vi "resonant.scan.engine.8or12kHz5ch_MD.vi"() -> ()   [LabVIEW 2012]
uses:
  <vilib>/Utility/VariantDataType/Type.ctl
  GFG/GFGbooleanGet.vi
  GFG/GFGnumericGet.vi
  GFG/GFGfpRefGet.vi
  <vilib>/Utility/error.llb/Error Cluster From Error Code.vi
  <vilib>/RVI Host/nirviSupport.llb/nirviErrorClusterFromErrorCode.vi
  <vilib>/rvi/errors/niLvFpgaAdjustHostInterfaceError.vi
  <vilib>/FPGAPlugInAG/PXIe-7962R/niLvFpga_Abort_PXIe-7962R.vi
  <vilib>/FPGAPlugInAG/PXIe-7962R/niLvFpga_Close_PXIe-7962R.vi
  <vilib>/rvi/interface/nirviMethod/nirviMethod.xnode
  FPGA/current bitfiles/4chresonancescan_PXIe-7962R_5ch8or12kHzreson_gAN2W9JJOBI.lvbitx
  <vilib>/rvi/interface/nirviCloseFPGA/nirviCloseFPGA.xnode
  GFG/GFG library.lvlib
  <vilib>/Utility/VariantDataType/VariantType.lvlib
  <vilib>/rvi/errors/niLvFpgaMergeErrorWithErrorCode.vi
  <vilib>/FPGAPlugInAG/PXIe-7962R/niLvFpga_AcknowledgeIrq_PXIe-7962R.vi
  <vilib>/rvi/interface/nirviMethod/StockFPGA_InlinedMethodWaitForSingleIRQ.vi
  <vilib>/FPGAPlugInAG/PXIe-7962R/niLvFpga_WaitOnIrq_PXIe-7962R.vi
  <vilib>/FPGAPlugInAG/PXIe-7962R/niLvFpga_ReadFifo_PXIe-7962R.vi
panel:
  out "x/y":dbl format="%#_6f"
  out "max Elements Remaining 2":u32
  out "Array":i16[][][](array[numeric])
  out "size(s)":i32[](array[numeric])
  out "Elements Remaining":u32
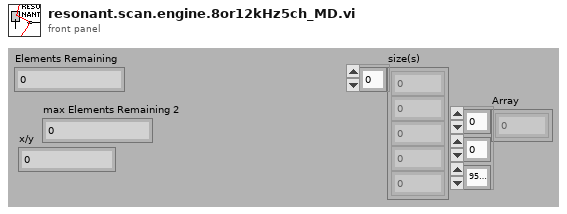
[diagram p1: front panel]
types:
  T1 = enum8{"Enabled", "Disabled", "Disabled and Grayed Out"}
  T2 = cluster{"WaveformChartRef":refnum<vi>, "DigitalRef":refnum<vi>, "ArrayRef":refnum<vi>, "TabControlRef":refnum<vi>, "EnumRef":refnum<vi>, "RingRef":refnum<vi>, "BooleanRef":refnum<vi>, "KnobRef":refnum<vi>, "SlideRef":refnum<vi>, "PathRef":refnum<vi>, "StringRef":refnum<vi>, "ComboBox":refnum<vi>, "WaveformGraphRef":refnum<vi>}
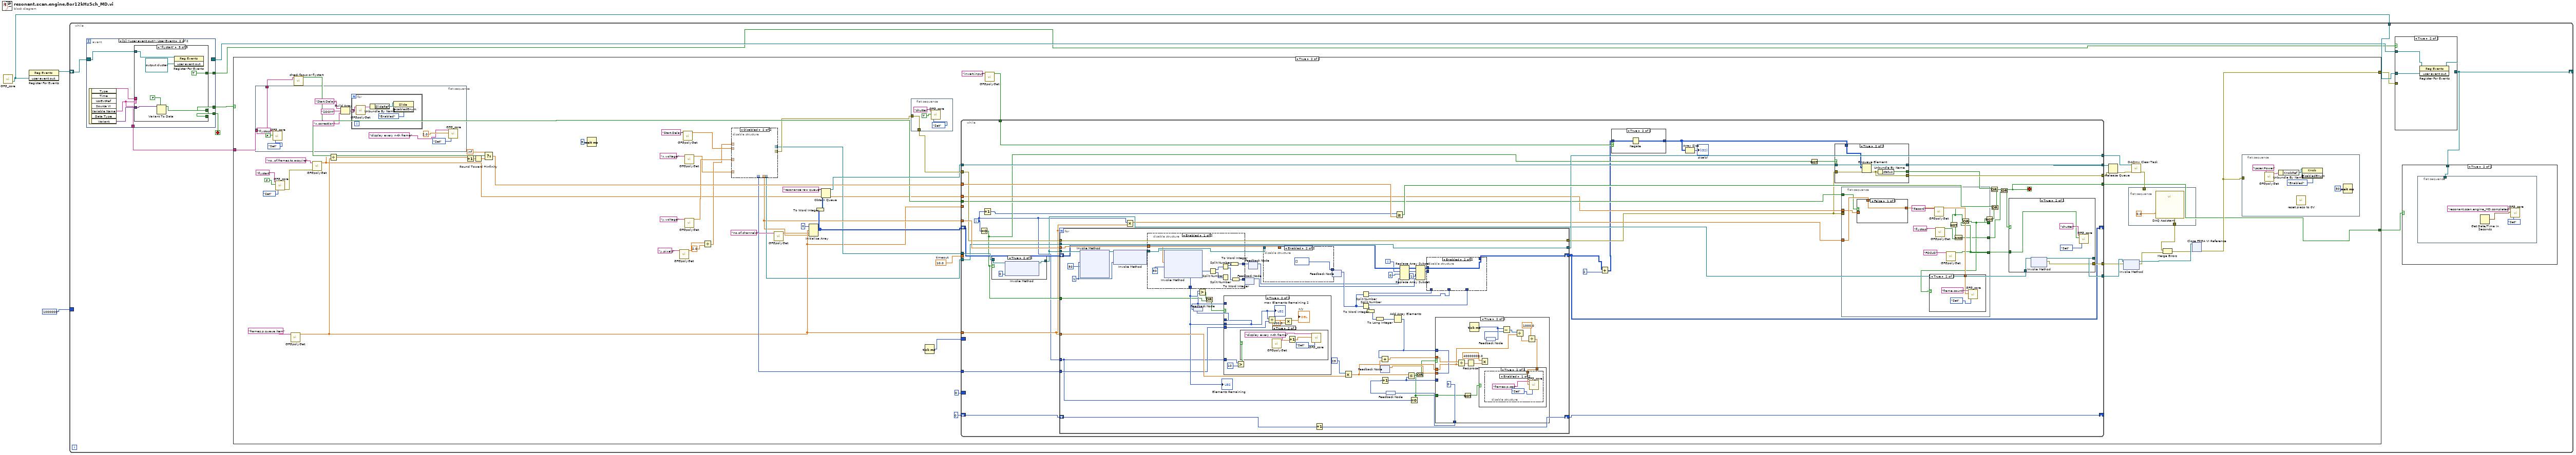
[diagram p0: block diagram]
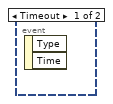
[diagram p4: hidden frame]
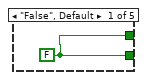
[diagram p5: hidden frame]
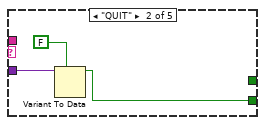
[diagram p6: hidden frame]
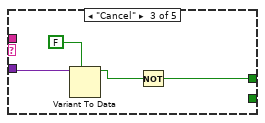
[diagram p7: hidden frame]
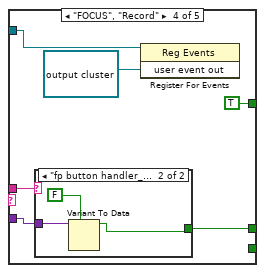
[diagram p8: hidden frame]
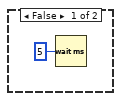
[diagram p10: hidden frame]
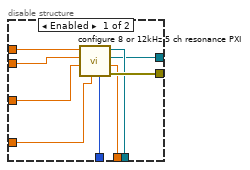
[diagram p11: hidden frame]
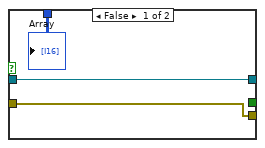
[diagram p12: hidden frame]
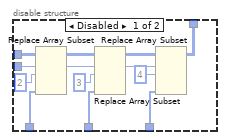
[diagram p13: hidden frame]
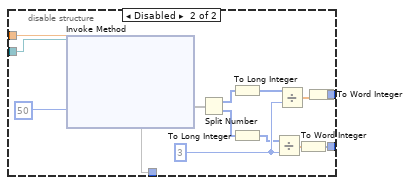
[diagram p14: hidden frame]
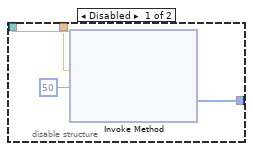
[diagram p15: hidden frame]
diagram:
  n1 = call "GFG_core.vi"() -> ("user event out"=w2:refnum<user-event>)  [unwired: 13 in, 6 out]
  n2 = register-events(w2) -> (reference out=w3:refnum<event-registration>)  [unwired: 2 in, 1 out]
  n3 = while {
    shift-right: [w4] -> _
    shift-left: w3 -> [w11]
    tunnel: w2 -> [w10]
    border: u32 1000000 ("Elements Remaining") -> [_]
    stop <- w12 stop-if-true
    n4 = event shown="[1] <user event out>: User Event" {
      selector: w11 -> [_ w24]
      dyn-events: [_ _] -> w8
      timeout: _ -> [_ _]
      tunnel: [_ w28] -> w13
      tunnel: [_ w27] -> w12
      tunnel: [_ w23] -> w7
      tunnel: [_ w22] -> w6
      event Timeout {
        n5 = event-data() -> ()  [unwired: 1 in, 2 out]
      }
      event User Event {
        n6 = event-data() -> ("Source VI"=w25:string, "Variable Name"=w22:string, "Variant"=w26:variant)  [unwired: 1 in, 4 out]
        n7 = case shown="\"flystart\"" w22 {
          tunnel: [w29 _ w33 w41 w46] -> w28
          tunnel: [w29 w30 _ _ _] -> w27
          tunnel: w26 -> [_ w32 w35 w42 w50]
          tunnel: w25 -> [_ _ _ w40 _]
          tunnel: w24 -> [_ _ _ w38 w47]
          tunnel: [_ _ _ TRUE TRUE] -> w23
          frame "False", Default {
            w29 = FALSE ("NewVal")
          }
          frame "QUIT" {
            n8 = Variant To Data(type=FALSE ("NewVal"), Variant=w32) -> (data=w30:bool)  [unwired: 1 in, 1 out]
          }
          frame "Cancel" {
            n9 = Variant To Data(type=FALSE ("NewVal"), Variant=w35) -> (data=w34:bool)  [unwired: 1 in, 1 out]
            n10 = Not(x=w34) -> (.not. x?=w33:bool)
          }
          frame "FOCUS", "Record" {
            n11 = case shown="\"fp button handler_MD.vi\"" w40 {
              tunnel: w42 -> [_ w44]
              tunnel: [_ w43] -> w41
              frame "False", Default {
              }
              frame "fp button handler_MD.vi" {
                n12 = Variant To Data(type=FALSE ("NewVal"), Variant=w44) -> (data=w43:bool)  [unwired: 1 in, 1 out]
              }
            }
            n13 = register-events(reference=w38, refnum<user-event> refnum ("user event out")) -> ()  [unwired: 1 in, 2 out]
          }
          frame "flystart" {
            n14 = Variant To Data(type=FALSE ("NewVal"), Variant=w50) -> (data=w46:bool)  [unwired: 1 in, 1 out]
            n15 = register-events(reference=w47, refnum<user-event> refnum ("user event out")) -> ()  [unwired: 1 in, 2 out]
          }
        }
      }
    }
    n16 = case shown="True" w13 {
      tunnel: [_ w88] -> w9
      tunnel: w6 -> [_ w56]
      tunnel: [_ w78] -> w5
      frame False {
        n17 = Wait (ms)(milliseconds to wait=u32 5) -> ()  [unwired: 1 out]
      }
      frame True {
        w109 = 10.0  # timeout
        n18 = flat-sequence {
          tunnel: w56 -> [w129]
          tunnel: [w129] -> w55
          frame #0 {
            n19 = call "GFG_core.vi"("Variable Name in"="flystop", "Variant in"=FALSE ("Boolean"), "Action"=enum16{"Init", "Set", "Get"}."Set") -> ()  [unwired: 10 in, 7 out]
            n20 = Build Array("Start.Delay" ("Variable Name in"), "ZOOM" ("Variable Name in"), "x.correction" ("Variable Name in")) -> (w124:string[])
            n21 = for {
              tunnel: w124 -> [w132] mode=indexing
              n22 = call-poly "GFGpolyGet.vi"("Variable Name in"=w132) -> ("output cluster"=w135:T2)  [unwired: 9 in, 1 out]
              n23 = Unbundle By Name(w135) -> ("SlideRef"=w133:refnum<vi>)
              n24 = property class="Slide"(reference=w133, "DisabledEnum"=T1."Enabled" ("Disabled")) -> ()  [unwired: 1 in, 2 out]
            }
            n25 = call "GFG_core.vi"("Variable Name in"="display every n-th frame" ("Tag in"), "Variant in"=2.0 ("Numeric"), "Action"=enum16{"Init", "Set", "Get"}."Set") -> ()  [unwired: 10 in, 7 out]
          }
        }
        n26 = call "GFG_core.vi"("Variable Name in"="flystart" ("Tag in"), "Variant in"=FALSE, "Action"=enum16{"Init", "Set", "Get"}."Set") -> ("error out"=w79:errorcluster)  [unwired: 10 in, 6 out]
        n27 = call-poly "GFGpolyGet.vi"("Variable Name in"="frames.p.queue.item" ("Tag in")) -> ("Numeric"=w61:dbl)  [unwired: 9 in, 1 out]
        n28 = call "check focus or flystart.vi"("x"=w55) -> ("x .or. y?"=w84:bool)  [unwired: 10 in]
        n29 = call-poly "GFGpolyGet.vi"("error in (no error)"=w79, "Variable Name in"="no..of.frames.to.acquire" ("Tag in")) -> ("Numeric"=w60:dbl)  [unwired: 8 in, 1 out]
        n30 = Divide(x=w60, y=w61) -> (x/y=w62:dbl)
        n31 = Increment(x=w62) -> (x+1=w57:dbl)
        n32 = Round Toward +Infinity(x=w57) -> (ceil(x): smallest int >= x=w59:dbl)
        n33 = Select(t=inf, s=w84, f=w59) -> (s? t:f=w85:dbl)
        n34 = Wait (ms)(milliseconds to wait=u32 5) -> ()  [unwired: 1 out]
        n35 = call-poly "GFGpolyGet.vi"("Variable Name in"="y.pixels" ("Tag in")) -> ("Numeric"=w103:dbl)  [unwired: 9 in, 1 out]
        n36 = call-poly "GFGpolyGet.vi"("Variable Name in"="Start.Delay" ("Tag in")) -> ("Numeric"=w75:dbl)  [unwired: 9 in, 1 out]
        n37 = call-poly "GFGpolyGet.vi"("Variable Name in"="x.voltage" ("Tag in")) -> ("Numeric"=w72:dbl)  [unwired: 9 in, 1 out]
        n38 = call-poly "GFGpolyGet.vi"("Variable Name in"="y.voltage" ("Tag in")) -> ("Numeric"=w74:dbl)  [unwired: 9 in, 1 out]
        n39 = Divide(x=w103, y=2.0 ("x")) -> (x/y=w73:dbl)
        n40 = disable-structure shown="Disabled" {
          disable-tunnel: w75 -> [w120 _]
          disable-tunnel: w74 -> [w119 _]
          disable-tunnel: w73 -> [w118 _]
          disable-tunnel: w72 -> [w117 _]
          disable-tunnel: [w116 _] -> w71
          disable-tunnel: [w115 _] -> w70
          disable-tunnel: [w114 _] -> w66
          disable-tunnel: [w112 _] -> w65
          disable-tunnel: [w113 _] -> w63
          frame Enabled {
            n41 = call "configure 8 or 12kHz 5 ch resonance PXI.vi"("x resonant zoom voltage"=w117, "y-voltage"=w119, "Start Delay (Ticks)"=w120, "lines (2pi) per frame"=w118) -> ("error out"=w116:errorcluster, "pixels per frame"=w114:dbl, "FPGA VI Reference Out"=w112:refnum<k20>, "AO task out"=w115:refnum<k21>, "Actual Depth 3"=w113:u32)  [unwired: 3 in]
          }
          frame Disabled {
          }
        }
        n42 = call-poly "GFGpolyGet.vi"("Variable Name in"="no.of.channels" ("Tag in")) -> ("Numeric"=w69:dbl)  [unwired: 9 in, 1 out]
        n43 = Initialize Array(i16 0, w61, w69, w66) -> (w95:i16[][][])
        n44 = To Word Integer(number=w95) -> (16bit integer=w53:i16[][][])
        n45 = Obtain Queue(name (unnamed)="resonance raw queue", element data type=w53) -> (queue out=w96:refnum<queue>)  [unwired: 3 in, 2 out]
        n46 = flat-sequence {
          tunnel: [w143] -> w105
          tunnel: w71 -> [w143]
          frame #0 {
            n47 = call "GFG_core.vi"("Variable Name in"="shutter" ("Tag in"), "Variant in"=TRUE, "Action"=enum16{"Init", "Set", "Get"}."Set") -> ()  [unwired: 10 in, 7 out]
          }
        }
        n48 = Tick Count (ms)() -> (millisecond timer value=w54:u32)
        n49 = call-poly "GFGpolyGet.vi"("Variable Name in"="invert.input" ("Tag in")) -> ("Boolean"=w106:bool)  [unwired: 10 in]
        n50 = while {
          tunnel: w70 -> [w173]
          tunnel: [w172] -> w111
          tunnel: [w183] -> w68
          tunnel: w96 -> [w186]
          tunnel: [w185] -> w110
          tunnel: w85 -> [w184]
          tunnel: w109 -> [_]
          tunnel: w105 -> [w174]
          tunnel: w106 -> [w181]
          tunnel: w65 -> [w177]
          tunnel: w66 -> [w175]
          tunnel: [w171] -> w94
          tunnel: [w170] -> w92
          tunnel: w84 -> [w169]
          tunnel: w60 -> [w168]
          tunnel: [w163] -> w78
          shift-right: [w149] -> _
          shift-left: w95 -> [w176]
          tunnel: w61 -> [w155]
          tunnel: w61 -> [_]
          border: 0 ("x+y") -> [_]
          tunnel: w63 -> [w157]
          shift-right: [w152] -> _
          shift-left: 0 ("x+y") -> [w153]
          border: w54 -> [_]
          i -> [w151]
          stop <- w163 stop-if-true
          n51 = Equal To 0?(x=w151) -> (x = 0?=w158:bool)
          n52 = Increment(x=w151) -> (x+1=w154:i32)
          n53 = case shown="True" w158 {
            tunnel: w177 -> [w322 w325]
            tunnel: [w322 w324] -> w162
            frame False {
            }
            frame True {
              n54 = xnode "Invoke Method"("FPGA VI Reference In"=w325, "IRQ Number(s)"=0) -> ("FPGA VI Reference Out"=w324:refnum<k20>)  [unwired: 1 in, 1 out]
            }
          }
          n55 = for {
            N: w155 -> [_]
            tunnel: [w245] -> w159
            tunnel: w174 -> [w245]
            tunnel: w173 -> [w243]
            tunnel: w175 -> [w241]
            tunnel: w162 -> [w244]
            shift-right: [w235] -> w149
            shift-left: w176 -> [w239]
            tunnel: [w243] -> w172
            tunnel: w155 -> [w223]
            tunnel: w158 -> [w215]
            tunnel: w157 -> [w214]
            shift-right: [w212] -> w152
            shift-left: w153 -> [w213]
            tunnel: w151 -> [w205]
            i -> [w234]
            w211 = 1 ("IRQ Number(s)")
            n56 = xnode "Invoke Method"("FPGA VI Reference In"=w244, "IRQ Number(s)"=w211, "Timeout (ms)"=50) -> ("FPGA VI Reference Out"=w210:refnum<k20>)  [unwired: 1 in, 3 out]
            n57 = xnode "Invoke Method"("FPGA VI Reference In"=w210, "IRQ Number(s)"=w211) -> ("FPGA VI Reference Out"=w242:refnum<k20>)  [unwired: 1 in, 1 out]
            n58 = disable-structure shown="Enabled" {
              disable-tunnel: w242 -> [w268 w278]
              disable-tunnel: w241 -> [w267 w277]
              disable-tunnel: [w266 w271] -> w219
              disable-tunnel: [w259 w273] -> w199
              disable-tunnel: [w258 w272] -> w198
              frame Enabled {
                n59 = xnode "Invoke Method"("FPGA VI Reference In"=w268, "Number of Elements"=w267, "Timeout (ms)"=50) -> ("Data"=w264:u64[], "Elements Remaining"=w266:u32)  [unwired: 1 in, 2 out]
                n60 = Split Number(x=w264) -> (hi(x)=w263:u32[], lo(x)=w262:u32[])
                n61 = Split Number(x=w263) -> (hi(x)=w261:u16[], lo(x)=w260:u16[])
                n62 = Split Number(x=w262) -> ()  [unwired: 2 out]
                n63 = To Word Integer(number=w261) -> (16bit integer=w259:i16[])
                n64 = To Word Integer(number=w260) -> (16bit integer=w258:i16[])
              }
              frame Disabled {
                w275 = 3
                n65 = xnode "Invoke Method"("FPGA VI Reference In"=w278, "Number of Elements"=w277, "Timeout (ms)"=50) -> ("Data"=w282:void[], "Elements Remaining"=w271)  [unwired: 1 in, 2 out]
                n66 = Split Number(x=w282) -> (hi(x)=w280:u16[], lo(x)=w279:u16[])
                n67 = To Long Integer(number=w280) -> (32bit integer=w276:i32[])
                n68 = To Long Integer(number=w279) -> (32bit integer=w269:i32[])
                n69 = Divide(x=w269, y=w275) -> (x/y=w270:dbl[])
                n70 = Divide(x=w276, y=w275) -> (x/y=w274:dbl[])
                n71 = To Word Integer(number=w270) -> (16bit integer=w272:i16[])
                n72 = To Word Integer(number=w274) -> (16bit integer=w273:i16[])
              }
            }
            "Elements Remaining" <- w219
            n73 = feedback #1() -> (w217:u32)
            n74 = Greater?(x=w219, y=w217) -> (0:w220:bool)
            n75 = Or(x=w220, y=w215) -> (x .or. y?=w216:bool)
            n76 = case shown="True" w216 {
              tunnel: w219 -> [_ w296]
              tunnel: [w288 w296] -> w218
              tunnel: w217 -> [w288 _]
              tunnel: w214 -> [_ w295]
              tunnel: w205 -> [_ w291]
              frame False {
              }
              frame True {
                n77 = Greater?(x=w291, y=10) -> (0:w289:bool)
                n78 = case shown="True" w289 {
                  frame False {
                  }
                  frame True {
                    w299 = "display every n-th frame" ("Tag in")
                    n79 = call-poly "GFGpolyGet.vi"("Variable Name in"=w299) -> ("Numeric"=w298:dbl)  [unwired: 9 in, 1 out]
                    n80 = Increment(x=w298) -> (x+1=w297:dbl)
                    n81 = call "GFG_core.vi"("Variable Name in"=w299, "Variant in"=w297, "Action"=enum16{"Init", "Set", "Get"}."Set") -> ()  [unwired: 10 in, 7 out]
                  }
                }
                n82 = Divide(x=w296, y=w295) -> (x/y=w294:dbl)
                n83 = Multiply(x=w294, y=100.0) -> (x*y=→"x/y":dbl)
                "max Elements Remaining 2" <- w296
              }
            }
            n84 = feedback-in #1(w218) -> ()
            n85 = feedback-in #2(w198) -> ()
            n86 = feedback #2() -> (w197:i16[])  [unwired: 1 in]
            n87 = feedback-in #3(w199) -> ()
            n88 = feedback #3() -> (w196:i16[])  [unwired: 1 in]
            n89 = disable-structure shown="Enabled" {
              disable-tunnel: w242 -> [w285 _]
              disable-tunnel: w241 -> [w284 _]
              disable-tunnel: [w283 u32[] [] ("lo(x)")] -> w240
              frame Disabled {
                n90 = xnode "Invoke Method"("FPGA VI Reference In"=w285, "Number of Elements"=w284, "Timeout (ms)"=50) -> ("Data"=w283:u32[])  [unwired: 1 in, 3 out]
              }
              frame Enabled {
              }
            }
            n91 = Increment(x=w213) -> (x+1=w212:i32)
            n92 = feedback-in #4(w240) -> ()
            n93 = feedback #4() -> (w200:u32[])  [unwired: 1 in]
            n94 = Multiply(x=u32 25, y=w223) -> (x*y=w222:dbl)
            n95 = Split Number(x=w200) -> (hi(x)=w203:u16[], lo(x)=w202:u16[])
            n96 = Split Number(x=w200) -> (hi(x)=w201:u16[], lo(x)=w221:u16[])
            n97 = To Word Integer(number=w221) -> (16bit integer=w207:i16[])
            n98 = To Long Integer(number=w207) -> (32bit integer=w228:i32[])
            n99 = feedback #5() -> (w232:dbl)  [unwired: 1 in]
            n100 = feedback #6() -> (w227:i32)
            n101 = Increment(x=w227) -> (x+1=w230:i32)
            n102 = Add Array Elements(numeric array=w228) -> (sum=w208:i32)
            n103 = Add(x=w208, y=w232) -> (x+y=w226:dbl)
            n104 = Replace Array Subset(array=w239, new element=w196, index (dim 0)=w234, index (dim 1)=0 ("disabled index (row)")) -> (w237:i16[][][])  [unwired: 1 in]
            n105 = Less Or Equal?(x=w222, y=w230) -> (x <= y?=w229:bool)
            n106 = Equal To 0?(x=w205) -> (x = 0?=w204:bool)
            n107 = Or(x=w204, y=w229) -> (x .or. y?=w206:bool)
            n108 = Replace Array Subset(array=w237, new element=w197, index (dim 0)=w234, index (dim 1)=1 ("disabled index (col)")) -> (w236:i16[][][])  [unwired: 1 in]
            n109 = disable-structure shown="Enabled" {
              disable-tunnel: w236 -> [w256 w257]
              disable-tunnel: [w253 w257] -> w235
              disable-tunnel: w234 -> [w252 _]
              disable-tunnel: w203 -> [w248 _]
              disable-tunnel: w202 -> [w247 _]
              disable-tunnel: w201 -> [w246 _]
              frame Disabled {
                n110 = Replace Array Subset(array=w256, new element=w248, index (dim 0)=w252, index (dim 1)=2 ("disabled index (col)")) -> (w255:i16[][][])  [unwired: 1 in]
                n111 = Replace Array Subset(array=w255, new element=w247, index (dim 0)=w252, index (dim 1)=3 ("disabled index (col)")) -> (w254:i16[][][])  [unwired: 1 in]
                n112 = Replace Array Subset(array=w254, new element=w246, index (dim 0)=w252, index (dim 1)=4 ("disabled index (row)")) -> (w253:i16[][][])  [unwired: 1 in]
              }
              frame Enabled {
              }
            }
            n113 = case shown="True" w206 {
              tunnel: w230 -> [w302 _]
              tunnel: [w302 0 ("x+y")] -> w231
              tunnel: w208 -> [_ w312]
              tunnel: w222 -> [_ w308]
              tunnel: w226 -> [w301 w313]
              tunnel: [w301 w312] -> w225
              tunnel: w204 -> [_ w304]
              frame False {
              }
              frame True {
                n114 = Divide(x=w313, y=w308) -> (x/y=w316:dbl)
                n115 = Not(x=w304) -> (.not. x?=w303:bool)
                n116 = Reciprocal(x=w316) -> (1/x=w315:dbl)
                n117 = Tick Count (ms)() -> (millisecond timer value=w311:u32)
                n118 = Multiply(x=40000000.0, y=w315) -> ()  [unwired: 1 out]
                n119 = feedback #7() -> (w310:u32)
                n120 = feedback-in #7(w311) -> ()
                n121 = Subtract(x=w311, y=w310) -> (x-y=w309:u32)
                n122 = Divide(x=w309, y=w308) -> (x/y=w307:dbl)
                n123 = Divide(x=1000.0, y=w307) -> (x/y=w305:dbl)
                n124 = case shown="True" w303 {
                  tunnel: w305 -> [_ w318]
                  frame False {
                  }
                  frame True {
                    n125 = disable-structure shown="Enabled" {
                      disable-tunnel: w318 -> [w319 _]
                      frame Enabled {
                        n126 = call "GFG_core.vi"("Variable Name in"="frames.p.sec", "Variant in"=w319, "Action"=enum16{"Init", "Set", "Get"}."Set") -> ()  [unwired: 10 in, 7 out]
                      }
                      frame Disabled {
                      }
                    }
                  }
                }
              }
            }
            n127 = feedback-in #5(w225) -> ()
            n128 = feedback-in #6(w231) -> ()
          }
          n129 = Multiply(x=w151, y=w155) -> (x*y=w156:dbl)
          n130 = Greater Or Equal?(x=w154, y=w184) -> (x >= y?=w179:bool)
          n131 = Add(x=w149, y=i16 2 ("millisecond timer value")) -> (x+y=w147:i16[][][])
          n132 = case shown="True" w181 {
            tunnel: [w326 w328] -> w150
            tunnel: w147 -> [w326 w327]
            frame False {
            }
            frame True {
              n133 = Negate(x=w327) -> (-x=w328:i16[][][])
            }
          }
          n134 = Array Size(array=w150) -> (size(s)=→"size(s)":i32[])
          n135 = Not(x=w158) -> (.not. x?=w160:bool)
          n136 = case shown="True" w160 {
            tunnel: w150 -> [w187 w190]
            tunnel: w186 -> [w189 w195]
            tunnel: [w189 w194] -> w185
            tunnel: [w188 w193] -> w183
            tunnel: [_ w192] -> w180
            tunnel: w159 -> [w188 w191]
            frame False {
              "Array" <- w187
            }
            frame True {
              n137 = Enqueue Element(queue=w195, element=w190, error in (no error)=w191) -> (queue out=w194:refnum<queue>, error out=w193:errorcluster)  [unwired: 1 in, 1 out]
              n138 = Unbundle By Name(w193) -> ("status"=w192:bool)
            }
          }
          n139 = flat-sequence {
            tunnel: [w332] -> w166
            tunnel: w159 -> [_]
            tunnel: w156 -> [w339]
            tunnel: w169 -> [w337]
            tunnel: w168 -> [w336]
            tunnel: [w329] -> w165
            tunnel: [w330] -> w164
            frame #0 {
              n140 = case shown="False" w337 {
                tunnel: w336 -> [_ w348]
                tunnel: w339 -> [w345 w347]
                tunnel: [w345 w346] -> w338
                frame False {
                }
                frame True {
                  n141 = Quotient & Remainder(x=w347, y=w348) -> (x-y*floor(x/y)=w346:dbl)  [unwired: 1 out]
                }
              }
              n142 = call-poly "GFGpolyGet.vi"("Variable Name in"="Record") -> ("Boolean"=w333:bool)  [unwired: 10 in]
              n143 = call-poly "GFGpolyGet.vi"("Variable Name in"="flystop") -> ("Boolean"=w331:bool)  [unwired: 10 in]
              n144 = call-poly "GFGpolyGet.vi"("Variable Name in"="FOCUS") -> ("Boolean"=w332:bool)  [unwired: 10 in]
              n145 = Not(x=w333) -> (.not. x?=w334:bool)
              n146 = And(x=w334, y=w331) -> (x .and. y?=w330:bool)
              n147 = Or(x=w333, y=w332) -> (x .or. y?=w329:bool)
              n148 = case shown="True" w329 {
                tunnel: w338 -> [_ w342]
                frame False {
                }
                frame True {
                  n149 = call "GFG_core.vi"("Variable Name in"="frame.count", "Variant in"=w342, "Action"=enum16{"Init", "Set", "Get"}."Set") -> ()  [unwired: 10 in, 7 out]
                }
              }
            }
          }
          n150 = Not(x=w165) -> (.not. x?=w182:bool)
          n151 = Or(x=w179, y=w182) -> (x .or. y?=w178:bool)
          n152 = Or(x=w180, y=w178) -> (x .or. y?=w167:bool)
          n153 = Or(x=w167, y=w164) -> (x .or. y?=w163:bool)
          n154 = case shown="True" w163 {
            tunnel: w162 -> [w349 w353]
            tunnel: [w349 w352] -> w171
            tunnel: [_ w351] -> w170
            tunnel: w166 -> [_ w350]
            frame False {
            }
            frame True {
              n155 = xnode "Invoke Method"("FPGA VI Reference In"=w353) -> ("FPGA VI Reference Out"=w352:refnum<k20>, "error out"=w351:errorcluster)  [unwired: 1 in]
              n156 = call "GFG_core.vi"("Variable Name in"="shutter" ("Tag in"), "Variant in"=w350, "Action"=enum16{"Init", "Set", "Get"}."Set") -> ()  [unwired: 10 in, 7 out]
            }
          }
        }
        n157 = Release Queue(queue=w110, error in (no error)=w68) -> (error out=w108:errorcluster)  [unwired: 1 in, 2 out]
        n158 = xnode "Invoke Method"("FPGA VI Reference In"=w94, "error in"=w92) -> ("FPGA VI Reference Out"=w93:refnum<k20>, "error out"=w91:errorcluster)
        n159 = flat-sequence {
          tunnel: [w136] -> w90
          tunnel: w67 -> [_]
          frame #0 {
            n160 = call "DAQ Assistant"("data"=0.0) -> ("error out"=w136:errorcluster)  [unwired: 17 in, 1 out]
          }
        }
        n161 = call <vilib>:"DAQmx Clear Task.vi"("task in"=w111, "error in"=w108) -> ("error out"=w67:errorcluster)  [unwired: 13 in]
        n162 = Merge Errors(w90, w91) -> (w89:errorcluster)
        n163 = xnode "Close FPGA VI Reference"("FPGA VI Reference In"=w93, "error in"=w89) -> ("error out"=w88:errorcluster)
        n164 = flat-sequence {
          tunnel: w88 -> [_]
          frame #0 {
            n165 = call-poly "GFGpolyGet.vi"("Variable Name in"="Laser.Power") -> ("output cluster"=w142:T2)  [unwired: 9 in, 1 out]
            n166 = Unbundle By Name(w142) -> ("KnobRef"=w139:refnum<vi>)
            n167 = call "reset piezo to 0V.vi"() -> ()  [unwired: 11 in, 1 out]
            n168 = property class="Knob"(reference=w139, "DisabledEnum"=T1."Enabled" ("Disabled")) -> ()  [unwired: 1 in, 2 out]
            n169 = Wait (ms)(milliseconds to wait=u32 50) -> ()  [unwired: 1 out]
          }
        }
      }
    }
    n170 = case shown="True" w7 {
      tunnel: w10 -> [_ w21]
      tunnel: w9 -> [_ _]
      tunnel: [w18 w20] -> w4
      tunnel: w8 -> [w18 w19]
      frame False {
      }
      frame True {
        n171 = register-events(reference=w19, w21) -> (reference out=w20:refnum<event-registration>)  [unwired: 1 in, 1 out]
      }
    }
    n172 = case shown="True" w5 {
      tunnel: w4 -> [_ w14]
      frame False {
      }
      frame True {
        n173 = flat-sequence {
          tunnel: w14 -> [_]
          frame #0 {
            n174 = Get Date/Time In Seconds() -> (seconds since 1Jan1904=w15:timestamp)
            n175 = call "GFG_core.vi"("Variable Name in"="resonant.scan.engine_MD.completed", "Variant in"=w15, "Action"=enum16{"Init", "Set", "Get"}."Set") -> ()  [unwired: 10 in, 7 out]
          }
        }
      }
    }
  }
